vi "Start Flow (Specified Volume).vi"(6 "Reset Volume Counter (T)":bool=TRUE, 7 "Pump ID (0:A)":T2, 8 "error in (no error)":errorcluster, 9 "Direction (0: Aspirate)":T1, 10 "Volume (0 uL)":dbl, 11 "VISA resource in":refnum<visa-resource-name>) -> (0 "error out":errorcluster, 3 "VISA resource out":refnum<visa-resource-name>)   [LabVIEW 2015, in "Global FIA milliGAT.lvlib"]
doc: "Starts the pump to dispense the specified volume."
uses:
  Global FIA milliGAT.lvlib
  Utility/Pump Direction.ctl
  Private/Pump Parameter.ctl
  Utility/Pump Address.ctl
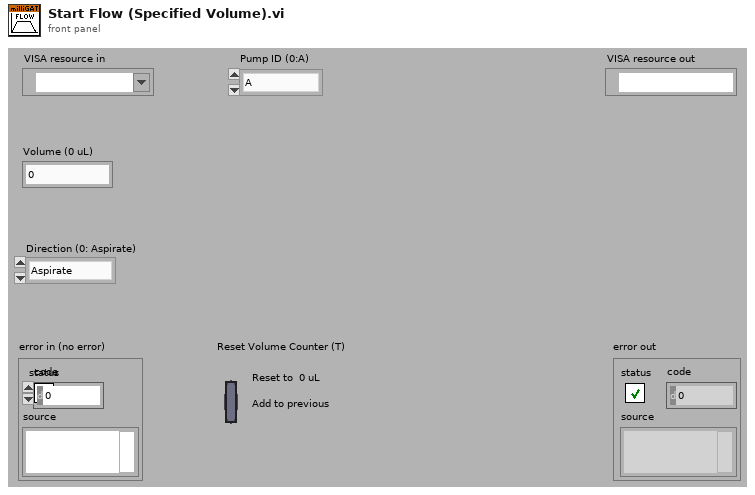
[diagram p1: front panel]
types:
  T1 = typedef "Global FIA milliGAT.lvlib/Pump Direction.ctl" = enum16{"Aspirate", "Dispense"}
  T2 = typedef "Global FIA milliGAT.lvlib/Pump Address.ctl" = enum16{"A", "B", "C", "D", "E", "F", "G", "H", "I", "J", "K", "L", "M", "N", "O", "P", "Q", "R", "S", "T", "U", "V", "W", "X", "Y", "Z", "a", "b", "c", "d", "e", "f", "g", "h", "i", "j", "k", "l", "m", "n", "o", "p", "q", "r", "s", "t", "u", "v", "w", "x", "y", "z", "0", "1", "2", "3", "4", "5", "6", "7", "8", "9"}
  T3 = typedef "Global FIA milliGAT.lvlib/Pump Parameter.ctl" = enum16{"Enabled", "EU", "EU Calibration Factor", "Fixed Asp or Disp", "Starting Position", "Starting Flow", "Peak Flow", "Flow Acceleration", "Flow Deceleration", "Session Volume", "Max Pressure", "Backlash (usteps)", "BL Calibration Factor", "BL Correction Enabled", "Min Flow", "Max Flow", "Min Acceleration", "Max Acceleration", "Service Volume", "Life Volume"}
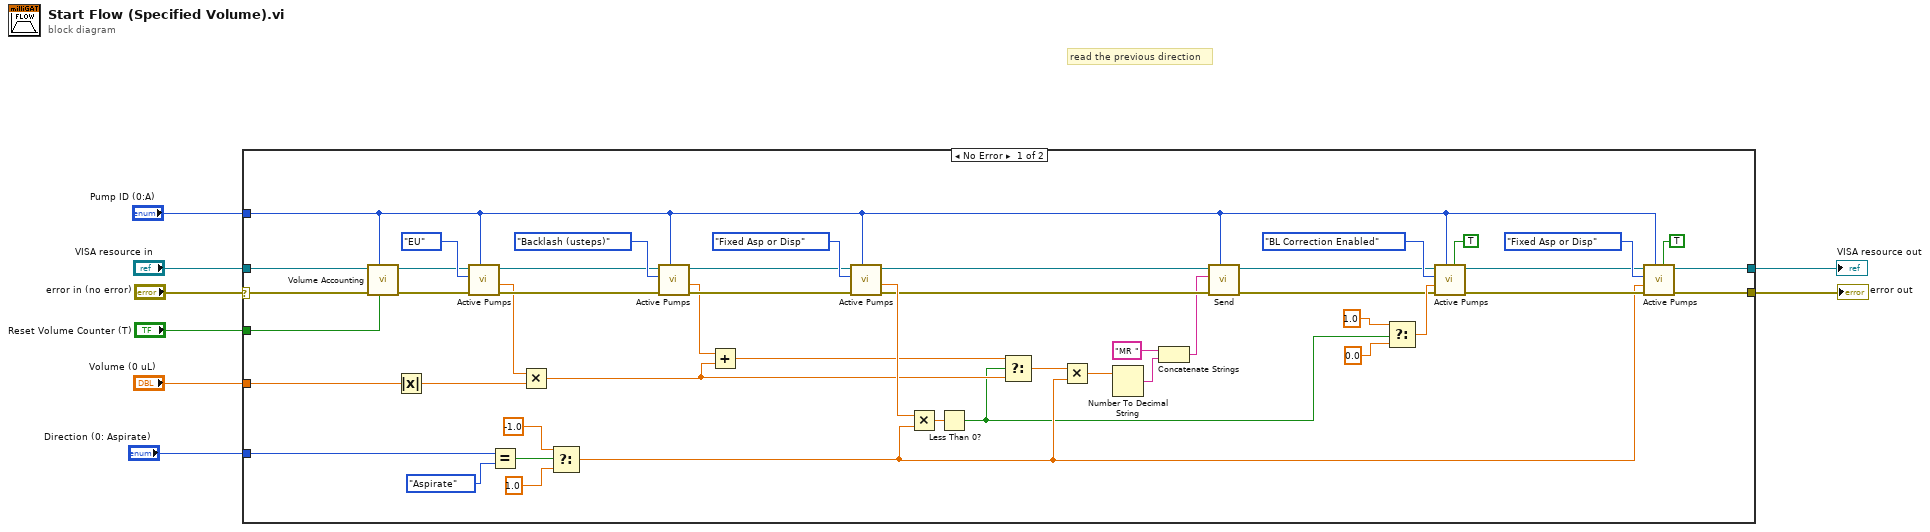
[diagram p0: block diagram]
diagram:
  # "read the previous direction"
  n1 = case shown="No Error" "error in (no error)" {
    selector: "error in (no error)" -> [w9 w58]
    tunnel: "Direction (0: Aspirate)" -> [w56 _]
    tunnel: "Volume (0 uL)" -> [w51 _]
    tunnel: "VISA resource in" -> [w49 w57]
    tunnel: "Reset Volume Counter (T)" -> [w48 _]
    tunnel: [w36 w57] -> w4
    tunnel: [w35 w58] -> w3
    tunnel: "Pump ID (0:A)" -> [w26 _]
    frame No Error {
      n2 = call "Volume Accounting.vi"("Reset Volume Counter (T)"=w48, "Pump ID (0:A)"=w26, "error in (no error)"=w9, "VISA resource in"=w49) -> ("error out"=w47:errorcluster, "VISA resource out"=w46:refnum<visa-resource-name>)  [unwired: 6 in]
      n3 = Absolute Value(x=w51) -> (abs(x)=w27:dbl)
      n4 = call "Active Pumps.vi"("Pump ID (0:A)"=w26, "error in (no error)"=w47, "Parameter"=Pump_Parameter."EU", "VISA resource in"=w46) -> ("error out"=w32:errorcluster, "Value out"=w28:dbl, "VISA resource out"=w31:refnum<visa-resource-name>)  [unwired: 4 in, 1 out]
      n5 = Equal?(x=w56, y=Pump_Direction."Aspirate") -> (x = y?=w54:bool)
      n6 = Multiply(x=w28, y=w27) -> (x*y=w21:dbl)
      n7 = Select(t=-1.0, s=w54, f=1.0) -> (s? t:f=w19:dbl)
      n8 = call "Active Pumps.vi"("Pump ID (0:A)"=w26, "error in (no error)"=w32, "Parameter"=Pump_Parameter."Backlash (usteps)", "VISA resource in"=w31) -> ("error out"=w29:errorcluster, "Value out"=w25:dbl, "VISA resource out"=w30:refnum<visa-resource-name>)  [unwired: 4 in, 1 out]
      n9 = Add(x=w25, y=w21) -> (x+y=w23:dbl)
      n10 = call "Active Pumps.vi"("Pump ID (0:A)"=w26, "error in (no error)"=w29, "Parameter"=Pump_Parameter."Fixed Asp or Disp", "VISA resource in"=w30) -> ("error out"=w18:errorcluster, "Value out"=w24:dbl, "VISA resource out"=w17:refnum<visa-resource-name>)  [unwired: 4 in, 1 out]
      n11 = Multiply(x=w24, y=w19) -> (x*y=w22:dbl)
      n12 = Less Than 0?(x=w22) -> (x < 0?=w10:bool)
      n13 = Select(t=w23, s=w10, f=w21) -> (s? t:f=w20:dbl)
      n14 = Multiply(x=w20, y=w19) -> (x*y=w15:dbl)
      n15 = Number To Decimal String(number=w15) -> (decimal integer string=w14:string)  [unwired: 1 in]
      n16 = Concatenate Strings("MR " ("string"), w14) -> (w13:string)
      n17 = call "Send.vi"("Pump ID (0:A)"=w26, "error in (no error)"=w18, "Command"=w13, "VISA resource in"=w17) -> ("error out"=w12:errorcluster, "VISA resource out"=w11:refnum<visa-resource-name>)  [unwired: 5 in, 1 out]
      n18 = Select(t=1.0 ("y"), s=w10, f=0.0) -> (s? t:f=w34:dbl)
      n19 = call "Active Pumps.vi"("Action (F:Read)"=TRUE, "Pump ID (0:A)"=w26, "error in (no error)"=w12, "Value in"=w34, "Parameter"=Pump_Parameter."BL Correction Enabled", "VISA resource in"=w11) -> ("error out"=w39:errorcluster, "VISA resource out"=w40:refnum<visa-resource-name>)  [unwired: 2 in, 2 out]
      n20 = call "Active Pumps.vi"("Action (F:Read)"=TRUE, "Pump ID (0:A)"=w26, "error in (no error)"=w39, "Value in"=w19, "Parameter"=Pump_Parameter."Fixed Asp or Disp", "VISA resource in"=w40) -> ("error out"=w35:errorcluster, "VISA resource out"=w36:refnum<visa-resource-name>)  [unwired: 2 in, 2 out]
    }
    frame Error {
    }
  }
  "VISA resource out" <- w4
  "error out" <- w3
